vi "Configure Session.vi"(8 "error in":errorcluster, 11 "Plugin in":refnum<class "Waterfall.lvclass">) -> (0 "error out":errorcluster, 3 "Plugin out":refnum<class "Waterfall.lvclass">)   [LabVIEW 2024, in "Waterfall.lvlib" / "Waterfall.lvclass"]
uses:
  Waterfall.lvclass
  C:/Program Files/National Instruments/LabVIEW 2024/vi.lib/FlexLogger/SDK/PluginSDK.lvlibp/PEFClasses/SDK/Plugin/Plugin.lvclass
  Waterfall Data.ctl
  <vilib>/Analysis/4window.llb/windowTd.ctl
  Waterfall.lvclass/Waterfall.ctl
  Waterfall Global.vi
  <vilib>/FlexLogger/SDK/PluginSDK.lvlibp/PEFClasses/SDK/Plugin/ParameterAccess/Read DBL.vi
  <vilib>/FlexLogger/SDK/PluginSDK.lvlibp/PEFClasses/SDK/Plugin/ParameterAccess/Read Enum.vi
  <vilib>/FlexLogger/SDK/PluginSDK.lvlibp/PEFClasses/SDK/Plugin/ParameterAccess/Read I32.vi
  <vilib>/FlexLogger/SDK/PluginSDK.lvlibp/PEFClasses/SDK/Plugin/Plugin.lvclass
  <vilib>/Analysis/NI_AALPro.lvlib
  <vilib>/Utility/LVLibp/NI_PackedLibraryUtility.lvlib
  C:/Program Files/National Instruments/LabVIEW 2024/vi.lib/FlexLogger/SDK/PluginSDK.lvlibp/PEFClasses/SDK/Processing Element/Processing Element.lvclass
  C:/Users/Administrator/Documents/LabVIEW Projects/FlexLogger IO Plug-ins/Waterfall/Waterfall.lvclass
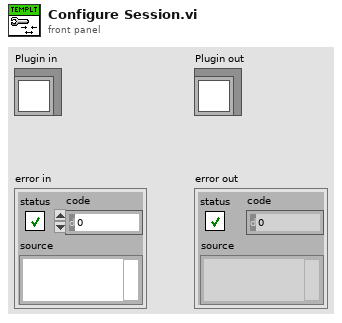
[diagram p1: front panel]
types:
  T1 = typedef "Waterfall.lvlib/Waterfall.lvclass/Waterfall Data.ctl" = cluster{"First Time":bool, "Show Waterfall Button Clicked":bool, "Data to Process":dbl, "Slice":dbl, "window":T2, "averaging parameters":cluster{"averaging mode":enum16{"No averaging", "Vector averaging", "RMS averaging", "Peak hold"}, "weighting mode":enum16{"Linear", "Exponential"}, "number of averages":u32}, "Waterfall VI Ref":refnum<vi>, "Signal":waveform(dbl)}
  T2 = typedef "NI_AALPro.lvlib/windowTd.ctl" = u32
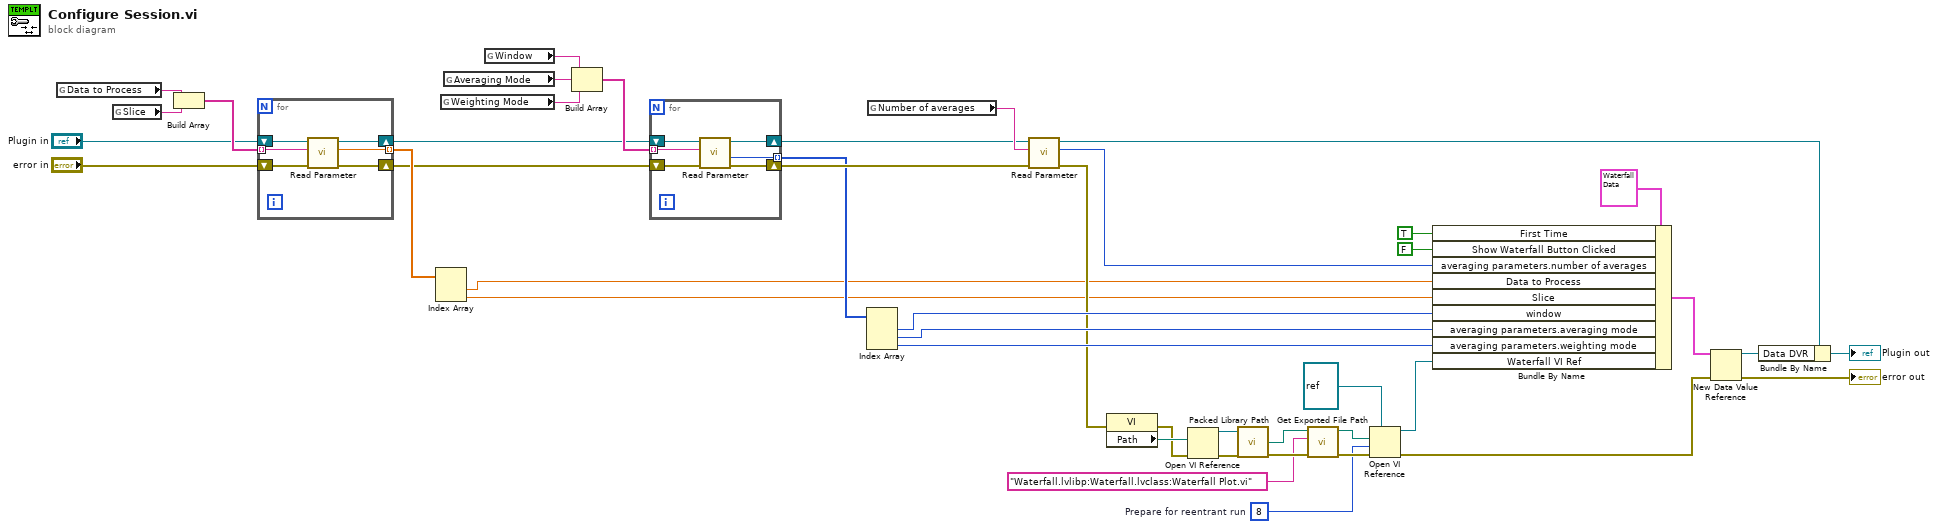
[diagram p0: block diagram]
diagram:
  w22 = 8  # Prepare for reentrant run
  n1 = global read "Waterfall Global.vi" "Data to Process"() -> (w12:string)
  n2 = global read "Waterfall Global.vi" "Slice"() -> (w11:string)
  n3 = Build Array(w12, w11) -> (w10:string[])
  n4 = for {
    shift-right: [w49] -> w3
    shift-left: "Plugin in" -> [w50]
    shift-right: [w47] -> w2
    shift-left: "error in" -> [w48]
    tunnel: [w45] -> w8 mode=indexing
    tunnel: w10 -> [w46] mode=indexing
    n5 = call-poly <vilib>:"Read Parameter.vi"("error in (no error)"=w48, "Name"=w46, "Plugin in"=w50) -> ("error out"=w47:errorcluster, "Value"=w45:dbl, "Plugin out"=w49:refnum<class "Waterfall.lvclass">)  [unwired: 5 in, 1 out]
  }
  n6 = Index Array(array=w8) -> (element #1=w5:dbl, element #2=w7:dbl)  [unwired: 2 in]
  n7 = global read "Waterfall Global.vi" "Weighting Mode"() -> (w38:string)
  n8 = global read "Waterfall Global.vi" "Averaging Mode"() -> (w39:string)
  n9 = global read "Waterfall Global.vi" "Window"() -> (w40:string)
  n10 = Build Array(w40, w39, w38) -> (w16:string[])
  n11 = for {
    shift-right: [w55] -> w15
    shift-left: w3 -> [w56]
    shift-right: [w53] -> w14
    shift-left: w2 -> [w54]
    tunnel: w16 -> [w52] mode=indexing
    tunnel: [w51] -> w13 mode=indexing
    n12 = call-poly <vilib>:"Read Parameter.vi"("error in (no error)"=w54, "Name"=w52, "Plugin in"=w56) -> ("error out"=w53:errorcluster, "Index"=w51:i32, "Plugin out"=w55:refnum<class "Waterfall.lvclass">)  [unwired: 4 in, 2 out]
  }
  n13 = Index Array(array=w13) -> (element #1=w37:i32, element #2=w36:i32, element #3=w35:i32)  [unwired: 3 in]
  n14 = global read "Waterfall Global.vi" "Number of averages"() -> (w33:string)
  n15 = call-poly <vilib>:"Read Parameter.vi"("error in (no error)"=w14, "Name"=w33, "Plugin in"=w15) -> ("error out"=w20:errorcluster, "Value"=w32:i32, "Plugin out"=w34:refnum<class "Waterfall.lvclass">)  [unwired: 5 in, 1 out]
  n16 = property class="VI"(error in=w20) -> (error out=w25:errorcluster, "Path"=w31:path)  [unwired: 1 in, 1 out]
  n17 = Open VI Reference(vi path=w31, error in (no error)=w25) -> (vi reference=w30:refnum<vi>, error out=w29:errorcluster)  [unwired: 4 in]
  n18 = call <vilib>:"Packed Library Path.vi"("error in (no error)"=w29, "vi reference"=w30) -> ("error out"=w27:errorcluster, "packed library path"=w28:path)  [unwired: 1 in, 1 out]
  n19 = call <vilib>:"Get Exported File Path.vi"("error in (no error)"=w27, "qualified name"="Waterfall.lvlibp:Waterfall.lvclass:Waterfall Plot.vi", "packed library path"=w28) -> ("error out"=w23:errorcluster, "path"=w24:path)  [unwired: 7 in]
  n20 = Open VI Reference(type specifier VI Refnum (for type only)=refnum<vi> refnum, vi path=w24, options=w22, error in (no error)=w23) -> (vi reference=w1:refnum<vi>, error out=w19:errorcluster)  [unwired: 2 in]
  n21 = Bundle By Name(cluster=T1 {"First Time"=FALSE, "Show Waterfall Button Clicked"=FALSE, "Data to Process"=0.0, "Slice"=0.0, "window"=0, "averaging parameters"={"averaging mode"=enum."No averaging", "weighting mode"=enum."Linear", "number of averages"=0}, "Waterfall VI Ref"=refnum, "Signal"={"t0"=timestamp(0 s since 1904-01-01), "dt"=1.0, "Y"=[]}} ("Data"), "First Time"=TRUE, "Show Waterfall Button Clicked"=FALSE ("Show Waterfall Window"), "averaging parameters.number of averages"=w32, "Data to Process"=w5, "Slice"=w7, "window"=w37, "averaging parameters.averaging mode"=w36, "averaging parameters.weighting mode"=w35, "Waterfall VI Ref"=w1) -> (w41:T1)
  n22 = New Data Value Reference(data value=w41, error in=w19) -> (data value reference=w4:refnum<data-value>, error out=→"error out":errorcluster)
  n23 = Bundle By Name(cluster=w34, "Data DVR"=w4) -> (→"Plugin out":refnum<class "Waterfall.lvclass">)
